vi "SmartMotor Wait.vi"(0 "reference in":refnum<class "SmartMotor.lvclass">, 4 "Number of Milliseconds to Wait":u32=100, 5 "error in (no error)":errorcluster) -> (14 "reference out":refnum<class "SmartMotor.lvclass">, 19 "error out":errorcluster)   [LabVIEW 2017, in "SmartMotor.lvclass"]
uses:
  SmartMotor.lvclass
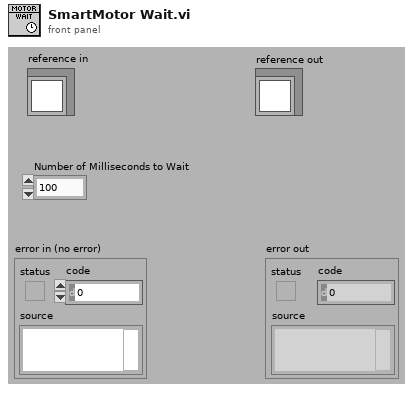
[diagram p1: front panel]
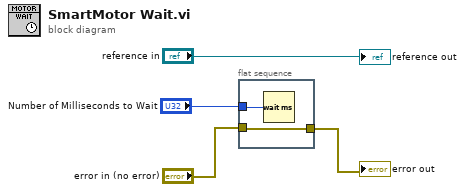
[diagram p0: block diagram]
diagram:
  n1 = flat-sequence {
    tunnel: "Number of Milliseconds to Wait" -> [w6]
    tunnel: "error in (no error)" -> [w5]
    tunnel: [w5] -> w3
    frame #0 {
      n2 = Wait (ms)(milliseconds to wait=w6) -> ()  [unwired: 1 out]
    }
  }
  "error out" <- w3
  "reference out" <- "reference in"
